vi "PrepareIESource.vi"   [LabVIEW 2020]
uses:
  <vilib>/Wiresmith Technology/G CLI/CLI Class/CLI.lvclass
  <userlib>/_OpenG.lib/file/file.llb/openg_file.lvlib
  <userlib>/_OpenG.lib/lvzip/lvzip.llb/ZLIB Open ZIP Mode__ogtk.ctl
  <vilib>/SLL Toolkit/SLL File IO/SLL File IO.lvlib
  <userlib>/_OpenG.lib/file/file.llb/Convert File Extension (Path)__ogtk.vi
  <userlib>/_OpenG.lib/lvzip/lvzip.llb/subVI/ZLIB Compress Directory (Path)__ogtk.vi
types:
  T1 = typedef "ZLIB Open ZIP Mode__ogtk.ctl" = enum16{"create new", "append to end", "append to archive"}
  T2 = enum32{"Invalid", "Standard", "Closed", "Hidden", "Minimized", "Maximized"}
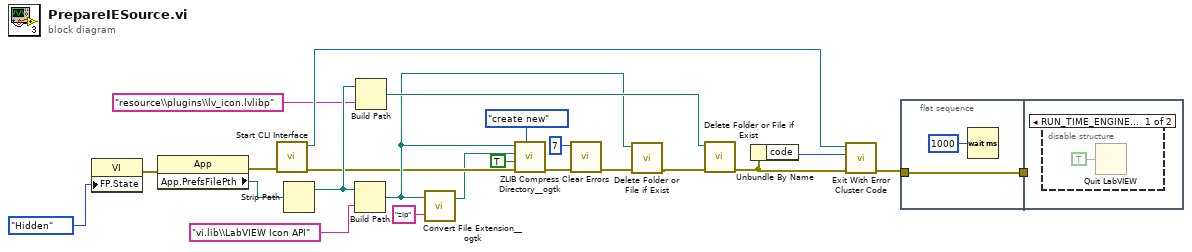
[diagram p0: block diagram]
diagram:
  n1 = property class="VI"("FP.State"=T2."Hidden" ("Front Panel Window:State")) -> (error out=w18:errorcluster)  [unwired: 2 in, 1 out]
  n2 = property class="App"(error in=w18) -> (error out=w17:errorcluster, "App.PrefsFilePth"=w16:path)  [unwired: 1 in, 1 out]
  n3 = call <vilib>:"Start CLI Interface.vi"("error in (no error)"=w17) -> ("error out"=w6:errorcluster, "CLI out"=w23:refnum<class "CLI.lvclass">)  [unwired: 7 in, 2 out]
  n4 = Strip Path(path=w16) -> (stripped path=w12:path)  [unwired: 1 out]
  n5 = Build Path(base path=w12, name or relative path="vi.lib\\LabVIEW Icon API" ("name")) -> (appended path=w7:path)
  n6 = Build Path(base path=w12, name or relative path="resource\\plugins\\lv_icon.lvlibp" ("name")) -> (appended path=w10:path)
  n7 = call-poly <userlib>:"Convert File Extension__ogtk.vi"("new ending (none)"="zip", "file name"=w7) -> ("new filename"=w4:path)  [unwired: 1 out]
  n8 = call-poly <userlib>:"ZLIB Compress Directory__ogtk.vi"("append (create new)"=ZLIB_Open_ZIP_Mode__ogtk."create new", "error in (no error)"=w6, "include subdirectories (F)"=TRUE, "archive name (root directory with .zip ending)"=w4, "root directory (file dialog)"=w7) -> ("error out"=w3:errorcluster)  [unwired: 4 in, 2 out]
  n9 = call <vilib>:"Clear Errors.vi"("error in (no error)"=w3, "specific error code to clear (0: all)"=7) -> ("error out"=w1:errorcluster)  [unwired: 4 in, 1 out]
  n10 = call <vilib>:"Delete Folder or File if Exist.vi"("error in (no error)"=w1, "Path"=w7) -> ("error out"=w8:errorcluster)  [unwired: 8 in, 1 out]
  n11 = call <vilib>:"Delete Folder or File if Exist.vi"("error in (no error)"=w8, "Path"=w10) -> ("error out"=w9:errorcluster)  [unwired: 8 in, 1 out]
  n12 = Unbundle By Name(w9) -> ("code"=w20:i32)
  n13 = call <vilib>:"Exit With Error Cluster Code.vi"("error in (no error)"=w9, "No Error Code (0)"=w20, "CLI in"=w23) -> ("error out"=w21:errorcluster)  [unwired: 8 in]
  n14 = flat-sequence {
    tunnel: w21 -> [w25]
    tunnel: [w25] -> w22
    tunnel: w22 -> [_]
    frame #0 {
      n15 = Wait (ms)(milliseconds to wait=u32 1000) -> ()  [unwired: 1 out]
    }
    frame #1 {
      n16 = disable-structure shown="RUN_TIME_ENGINE==True" {
        frame condition #0 {
          n17 = Quit LabVIEW(quit? (T)=TRUE) -> ()
        }
        frame condition #1 (active) {
        }
      }
    }
  }
